vi "sio getbaud.vi"(11 "port":i32) -> (3 "function return":i32)   [LabVIEW 2012, in "PCOMM.lvlib"]
doc: "long WINAPI sio_getbaud(int port);"
uses:
  PCOMM.lvlib
  #001 2018-09-10/Data/PCOMM.DLL
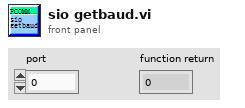
[diagram p1: front panel]
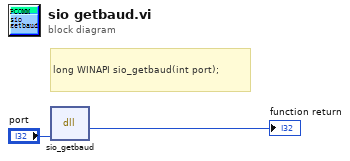
[diagram p0: block diagram]
diagram:
  # "long WINAPI sio_getbaud(int port);"
  n1 = dll-call lib="E:/ProJect/#008 ESDMonitor/#002 Labview/#001 2018-09-10/Data/PCOMM.*" fn="sio_getbaud"("port"="port") -> (→"function return":i32)  [unwired: 4 in, 2 out]
